vi "WiFi lab coordinator.vi"() -> ()   [LabVIEW 2014]
uses:
  VISA resource XBee.vi
  WiFi API Frame Type.ctl
  WiFi API Frame.ctl
  Protocol enum.ctl
panel:
  out "Port open":bool
  in  "Close serial comm":bool
  in  "Begin serial comm":bool
  in  "VISA resource in":refnum<visa-resource-name>
  out "Link Margin":u32
  out "Channel":u32
  out "Gateway IP":string
  out "Network Mask":string
  out "Destination IP Address":string
  out "Module IP Address":string
  out "Encryption":string
  out "SSID":string
  out "Connection Status":bool
  out "Association Information (AI)":string
  in  "Transparent response string":string
  in  "Transparent control string":string
  in  "Protocol":T1
  in  "Transparent mode enable":bool
  in  "API Response string":string
  in  "API Control string":string
  in  "Start session":bool
  in  "Destination port (hex)":u16=9750 step=1 format="%04x"
  in  "Source port (hex)":u16=2000 step=1 format="%04x"
  out "Source Port":u16
  out "Source IP":u8[](array[numeric])
  out "RF data":string
  # "Serial Port"
  # "Network Information"
  # "Session Configuration"
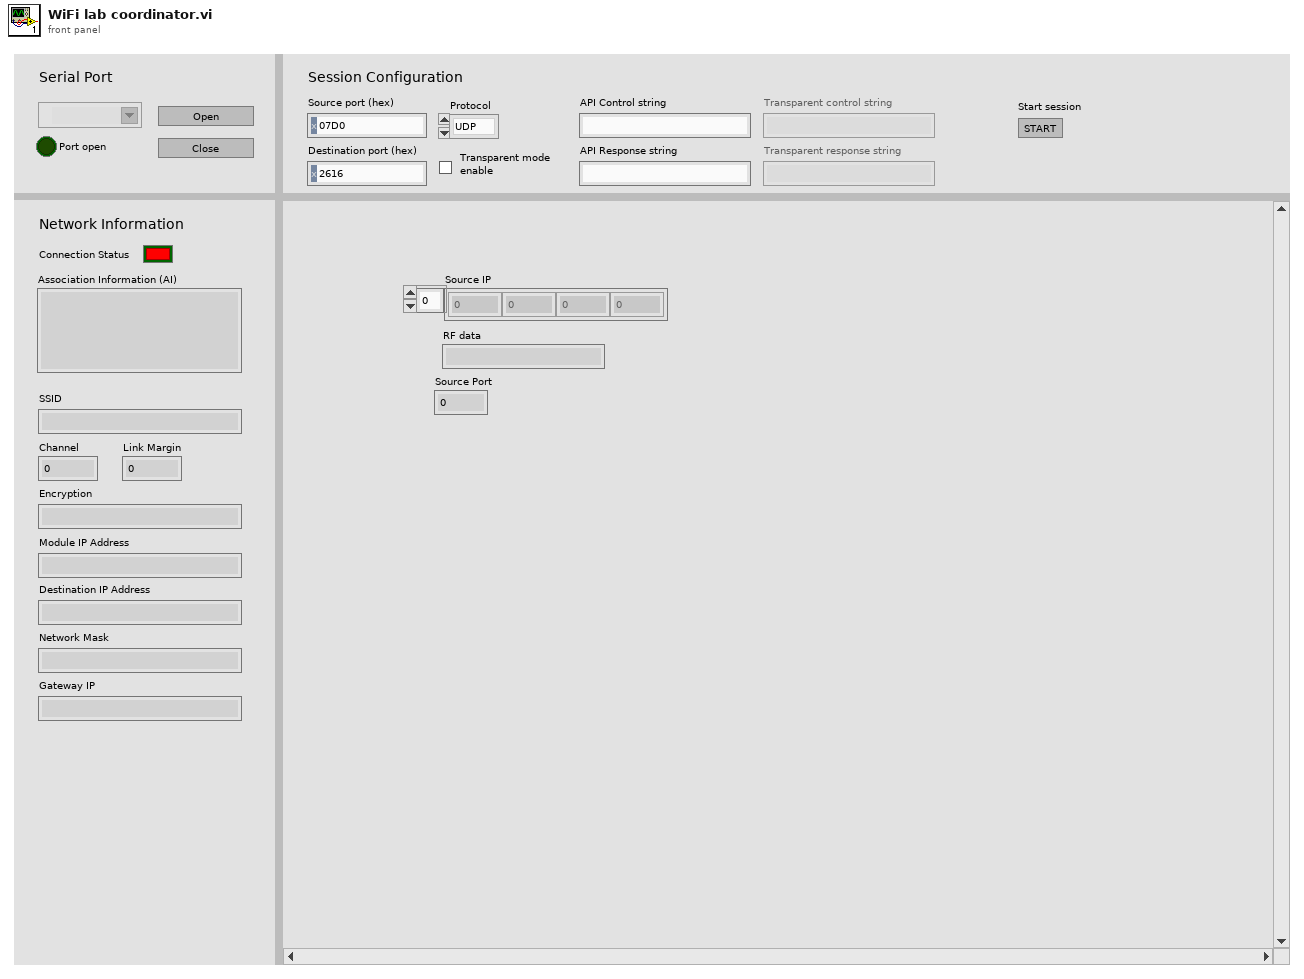
[diagram p1: front panel]
types:
  T1 = typedef "Protocol enum.ctl" = enum8{"UDP", "TCP"}
  T2 = typedef "WiFi API Frame.ctl" = cluster{"Length":u16, "Frame Type":T3, "Payload":u8[], "Checksum":u8}
  T3 = typedef "WiFi API Frame Type.ctl" = u8
  T4 = enum8{"Enabled", "Disabled", "Disabled and Grayed Out"}
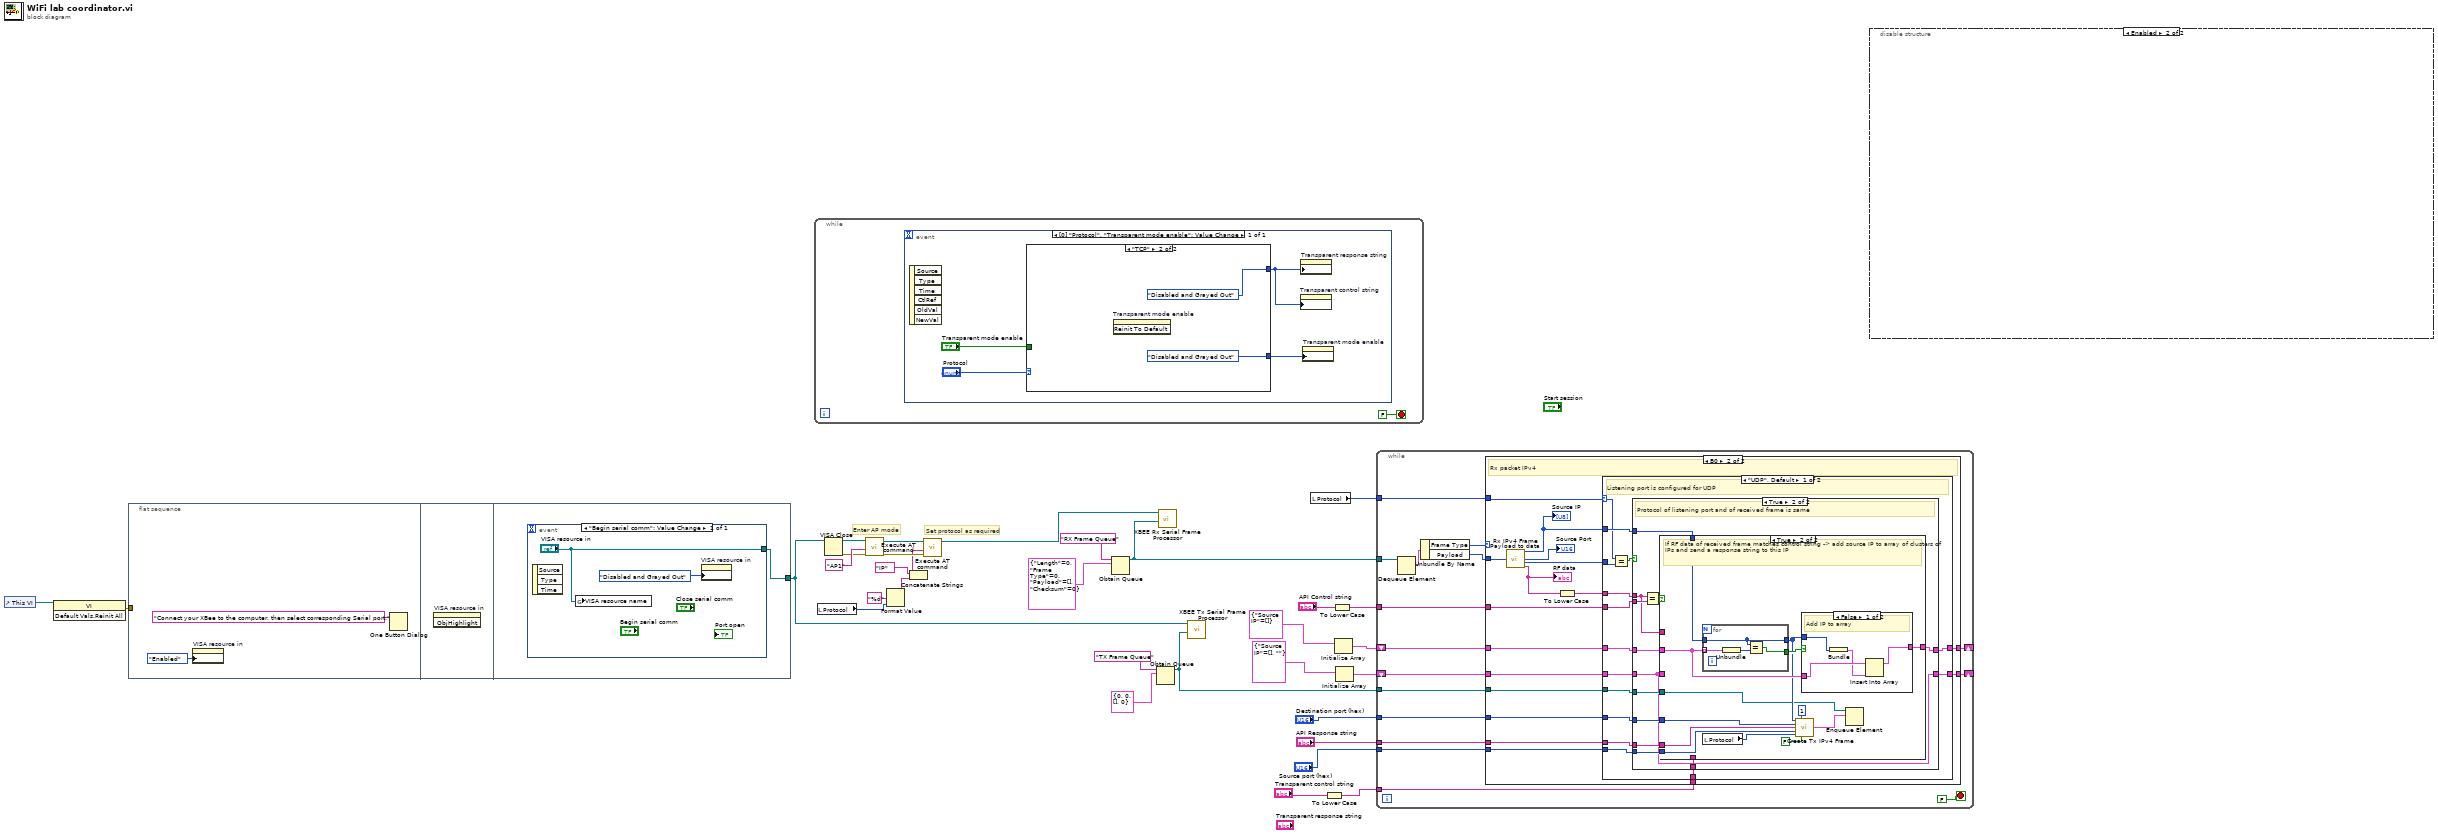
[diagram p0: block diagram]
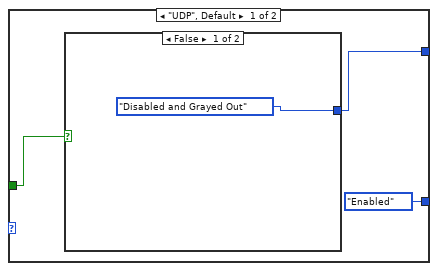
[diagram p2: hidden frame]
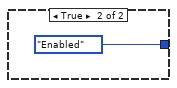
[diagram p3: hidden frame]
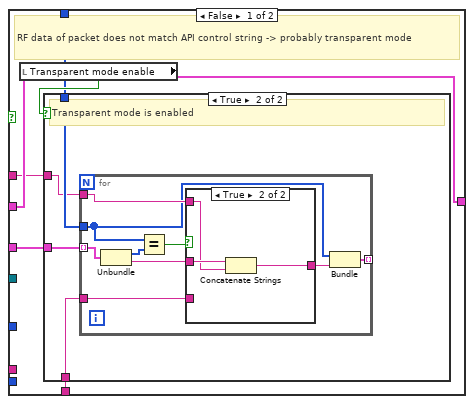
[diagram p6: hidden frame]
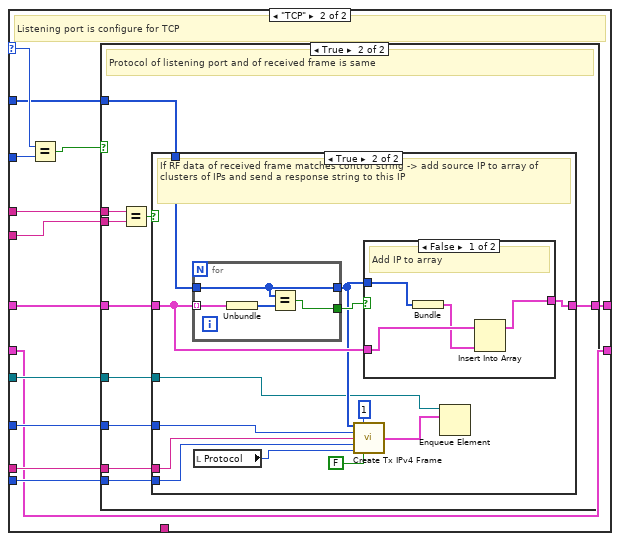
[diagram p10: hidden frame]
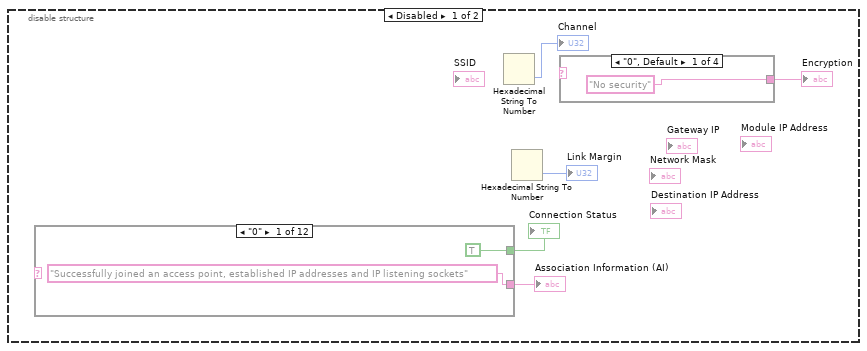
[diagram p14: hidden frame]
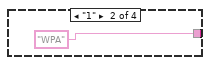
[diagram p15: hidden frame]
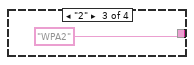
[diagram p16: hidden frame]
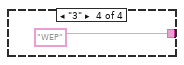
[diagram p17: hidden frame]
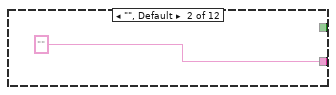
[diagram p18: hidden frame]
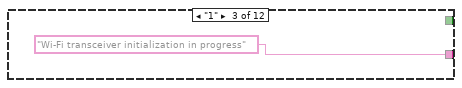
[diagram p19: hidden frame]
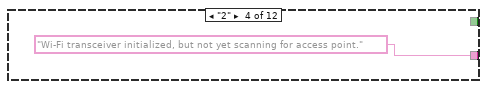
[diagram p20: hidden frame]
diagram:
  # "Set protocol as required"
  # "Enter AP mode"
  n1 = control-ref of="This VI"() -> (w31:refnum<vi>)
  n2 = invoke class="VI" method="Default Vals.Reinit All"(reference=w31) -> (error out=w30:errorcluster)  [unwired: 2 in, 2 out]
  n3 = flat-sequence {
    tunnel: w30 -> [_]
    tunnel: [w34] -> w11
    frame #0 {
      n4 = property on="VISA resource in" class="VISAName"("DisabledEnum"=T4."Enabled" ("Disabled")) -> ()  [unwired: 2 in, 2 out]
      n5 = One Button Dialog(message="Connect your XBee to the computer, then select corresponding Serial port.") -> ()  [unwired: 1 in, 1 out]
    }
    frame #1 {
      n6 = invoke on="VISA resource in" class="VISAName" method="ObjHighlight"() -> ()  [unwired: 3 in, 3 out]
    }
    frame #2 {
      n7 = event shown="[0] \"Begin serial comm\": Value Change" {
        selector: _ -> [_]
        dyn-events: _ -> [_]
        timeout: _ -> [_]
        tunnel: ["VISA resource in"] -> w34
        event "Begin serial comm": Value Change {
          n8 = event-data() -> ()  [unwired: 1 in, 3 out]
          n9 = global write "VISA resource XBee.vi" "VISA resource name"("VISA resource in") -> ()
          n10 = property on="VISA resource in" class="VISAName"("DisabledEnum"=T4."Disabled and Grayed Out" ("Disabled")) -> ()  [unwired: 2 in, 2 out]
        }
      }
    }
  }
  n11 = while {
    stop <- FALSE stop-if-true
    n12 = event shown="[0] \"Protocol\", \"Transparent mode enable\": Value Change" {
      selector: _ -> [_]
      dyn-events: _ -> [_]
      timeout: _ -> [_]
      event "Transparent mode enable": Value Change {
        n13 = event-data() -> ()  [unwired: 1 in, 6 out]
        n14 = case shown="\"TCP\"" "Protocol" {
          tunnel: [T4."Enabled" ("Disabled") T4."Disabled and Grayed Out" ("Disabled")] -> w38
          tunnel: [w42 T4."Disabled and Grayed Out" ("Disabled")] -> w39
          tunnel: "Transparent mode enable" -> [w43 _]
          frame "UDP", Default {
            n15 = case shown="False" w43 {
              tunnel: [T4."Disabled and Grayed Out" ("Disabled") T4."Enabled" ("Disabled")] -> w42
              frame False {
              }
              frame True {
              }
            }
          }
          frame "TCP" {
            n16 = invoke on="Transparent mode enable" class="Bool (strict)" method="Reinit To Default"() -> ()  [unwired: 3 in, 3 out]
          }
        }
        n17 = property on="Transparent control string" class="Str"("DisabledEnum"=w39) -> ()  [unwired: 2 in, 2 out]
        n18 = property on="Transparent response string" class="Str"("DisabledEnum"=w39) -> ()  [unwired: 2 in, 2 out]
        n19 = property on="Transparent mode enable" class="Bool (strict)"("DisabledEnum"=w38) -> ()  [unwired: 2 in, 2 out]
      }
    }
  }
  n20 = local read "Protocol"() -> (w3:T1)
  n21 = VISA Close(VISA resource name=w11) -> (error out=w8:errorcluster)  [unwired: 1 in]
  n22 = call "Execute AT command.vi"("error in (no error)"=w8, "AT Command"="AP1", "VISA resource in"=w11) -> ("error out"=w7:errorcluster, "VISA resource out"=w9:refnum<visa-resource-name>)  [unwired: 5 in, 1 out]
  n23 = Format Value(format string="%d", value (0)=w3) -> (output string=w2:string)  [unwired: 1 in]
  n24 = Concatenate Strings("IP" ("AT Command"), w2) -> (w5:string)
  n25 = call "Execute AT command.vi"("error in (no error)"=w7, "AT Command"=w5, "VISA resource in"=w9) -> ("VISA resource out"=w1:refnum<visa-resource-name>)  [unwired: 5 in, 2 out]
  n26 = Obtain Queue(name (unnamed)="RX Frame Queue", element data type=T2 {"Length"=0, "Frame Type"=0, "Payload"=[], "Checksum"=0} ("API Frame")) -> (queue out=w25:refnum<queue>)  [unwired: 3 in, 2 out]
  n27 = Obtain Queue(name (unnamed)="TX Frame Queue", element data type=T2 {"Length"=0, "Frame Type"=0, "Payload"=[], "Checksum"=0} ("API Frame")) -> (queue out=w19:refnum<queue>)  [unwired: 3 in, 2 out]
  n28 = call "XBEE Rx Serial Frame Processor.vi"("RX Frame Queue"=w25, "VISA Serial Port"=w1) -> ()  [unwired: 8 in, 2 out]
  n29 = call "XBEE Tx Serial Frame Processor.vi"("TX Frame Queue"=w19, "VISA Serial Port"=w11) -> ()  [unwired: 8 in, 2 out]
  n30 = local read "Protocol"() -> (w22:T1)
  n31 = To Lower Case(string="Transparent control string") -> (all lower case string=w12:string)
  n32 = To Lower Case(string="API Control string") -> (all lower case string=w23:string)
  n33 = Initialize Array(cluster{"Source IP":u8[]} {"Source IP"=[]}) -> (w21:cluster{"Source IP":u8[]}[])  [unwired: 1 in]
  n34 = Initialize Array(cluster{"Source IP":u8[], string} {"Source IP"=[], ""}) -> (w14:cluster{"Source IP":u8[], string}[])  [unwired: 1 in]
  n35 = while {
    tunnel: w25 -> [w64]
    tunnel: w23 -> [w59]
    tunnel: w22 -> [w58]
    shift-right: [w55] -> _
    shift-left: w21 -> [w57]
    tunnel: w19 -> [w56]
    tunnel: "Destination port (hex)" -> [w54]
    tunnel: "API Response string" -> [w53]
    tunnel: "Source port (hex)" -> [w52]
    shift-right: [w51] -> _
    shift-left: w14 -> [w49]
    tunnel: w12 -> [w50]
    stop <- FALSE stop-if-true
    n36 = Dequeue Element(queue=w64) -> (element=w63:T2)  [unwired: 2 in, 3 out]
    n37 = Unbundle By Name(w63) -> ("Frame Type"=w62:T3, "Payload"=w61:u8[])
    n38 = case shown="B0" w62 {
      tunnel: w61 -> [_ w83]
      tunnel: w59 -> [_ w78]
      tunnel: w58 -> [_ w80]
      tunnel: w57 -> [w66 w75]
      tunnel: w56 -> [_ w74]
      tunnel: [w66 w73] -> w55
      tunnel: w54 -> [_ w72]
      tunnel: w53 -> [_ w71]
      tunnel: w52 -> [_ w70]
      tunnel: w49 -> [w65 w69]
      tunnel: [w65 w68] -> w51
      tunnel: w50 -> [_ w67]
      frame 0, Default {
      }
      frame 176 {
        # "Rx packet IPv4"
        n39 = call "Rx IPv4 Frame Payload to data.vi"("Payload array"=w83) -> ("Source IP"=w76:u8[], "Source Port"=→"Source Port":u16, "Protocol"=w79:T1, "RF data"=w81:string)  [unwired: 10 in, 1 out]
        "RF data" <- w81
        "Source IP" <- w76
        n40 = To Lower Case(string=w81) -> (all lower case string=w77:string)
        n41 = case shown="\"UDP\", Default" w80 {
          selector: w80 -> [w87 w169]
          tunnel: w79 -> [w88 w170]
          tunnel: w78 -> [w95 w167]
          tunnel: w77 -> [w96 w166]
          tunnel: w76 -> [w90 w165]
          tunnel: w75 -> [w97 w164]
          tunnel: w74 -> [w94 w163]
          tunnel: [w98 w162] -> w73
          tunnel: w72 -> [w93 w161]
          tunnel: w71 -> [w92 w160]
          tunnel: w70 -> [w91 w159]
          tunnel: w69 -> [w86 w158]
          tunnel: [w85 w158] -> w68
          tunnel: w67 -> [w84 _]
          frame "UDP", Default {
            # "Listening port is configured for UDP"
            n42 = Equal?(x=w87, y=w88) -> (x = y?=w89:bool)
            n43 = case shown="True" w89 {
              tunnel: w95 -> [_ w112]
              tunnel: w96 -> [_ w102]
              tunnel: w90 -> [_ w109]
              tunnel: w97 -> [w100 w110]
              tunnel: w94 -> [_ w108]
              tunnel: [w100 w107] -> w98
              tunnel: w93 -> [_ w106]
              tunnel: w92 -> [_ w105]
              tunnel: w91 -> [_ w104]
              tunnel: w86 -> [w99 w103]
              tunnel: [w99 w103] -> w85
              tunnel: w84 -> [_ w101]
              frame False {
                # "Protocol of recieved frame does not match protocol of listening port. \nI know, right?"
              }
              frame True {
                # "Protocol of listening port and of received frame is same"
                n44 = Equal?(x=w102, y=w112) -> (x = y?=w111:bool)
                n45 = case shown="True" w111 {
                  tunnel: w110 -> [w117 w146]
                  tunnel: w109 -> [w115 w148]
                  tunnel: w108 -> [_ w137]
                  tunnel: [w117 w145] -> w107
                  tunnel: w106 -> [_ w143]
                  tunnel: w105 -> [_ w142]
                  tunnel: w104 -> [_ w141]
                  tunnel: w103 -> [w116 _]
                  tunnel: w102 -> [w114 _]
                  tunnel: w101 -> [w113 _]
                  frame False {
                    # "RF data of packet does not match API control string -> probably transparent mode"
                    n46 = local read "Transparent mode enable"() -> (w118:bool)
                    n47 = case shown="True" w118 {
                      tunnel: w116 -> [_ w122]
                      tunnel: w115 -> [_ w121]
                      tunnel: w114 -> [_ w120]
                      tunnel: w113 -> [_ w119]
                      frame False {
                        # "Transparent mode is disabled -> do nothing"
                      }
                      frame True {
                        # "Transparent mode is enabled"
                        n48 = for {
                          tunnel: w122 -> [w131] mode=indexing
                          tunnel: w121 -> [w125]
                          tunnel: w120 -> [w127]
                          tunnel: [w124] -> _ mode=indexing
                          tunnel: w119 -> [w123]
                          n49 = Unbundle(w131) -> ("Source IP"=w130:u8[], w128:string)
                          n50 = Equal?(x=w125, y=w130) -> (x = y?=w129:bool)
                          n51 = case shown="True" w129 {
                            tunnel: w128 -> [w132 w135]
                            tunnel: w127 -> [_ w134]
                            tunnel: [w132 w133] -> w126
                            tunnel: w123 -> [_ _]
                            frame False {
                            }
                            frame True {
                              n52 = Concatenate Strings(w135, w134) -> (w133:string)
                            }
                          }
                          n53 = Bundle("Source IP"=w125, w126) -> (w124:cluster{"Source IP":u8[], string})  [unwired: 1 in]
                        }
                      }
                    }
                  }
                  frame True {
                    # "If RF data of received frame matches control string -> add source IP to array of clusters of IPs and send a response string to this IP"
                    n54 = for {
                      tunnel: w146 -> [w157] mode=indexing
                      tunnel: w148 -> [w154]
                      tunnel: [w155] -> w147
                      tunnel: [w154] -> w144
                      n55 = Unbundle(w157) -> ("Source IP"=w156:u8[])
                      n56 = Equal?(x=w154, y=w156) -> (x = y?=w155:bool)
                    }
                    n57 = local read "Protocol"() -> (w140:T1)
                    n58 = call "Create Tx IPv4 Frame.vi"("Destination IP"=w144, "Frame ID"=u8 1, "Destination port"=w143, "RF data"=w142, "Source port"=w141, "Protocol"=w140, "Transmit options bitfield"=FALSE) -> ("TX IPv4 Frame"=w136:T2)  [unwired: 8 in]
                    n59 = case shown="False" w147 {
                      tunnel: w146 -> [w151 w153]
                      tunnel: w144 -> [w152 _]
                      tunnel: [w149 w153] -> w145
                      frame False {
                        # "Add IP to array"
                        n60 = Bundle("Source IP"=w152) -> (w150:cluster{"Source IP":u8[]})  [unwired: 1 in]
                        n61 = Insert Into Array(array=w151, new element=w150) -> (w149:cluster{"Source IP":u8[]}[])  [unwired: 1 in]
                      }
                      frame True {
                        # "IP already in array"
                      }
                    }
                    n62 = Enqueue Element(queue=w137, element=w136) -> ()  [unwired: 2 in, 3 out]
                  }
                }
              }
            }
          }
          frame "TCP" {
            # "Listening port is configure for TCP"
            n63 = Equal?(x=w169, y=w170) -> (x = y?=w168:bool)
            n64 = case shown="True" w168 {
              tunnel: w167 -> [_ w181]
              tunnel: w166 -> [_ w180]
              tunnel: w165 -> [_ w177]
              tunnel: w164 -> [w171 w178]
              tunnel: w163 -> [_ w176]
              tunnel: [w171 w175] -> w162
              tunnel: w161 -> [_ w174]
              tunnel: w160 -> [_ w173]
              tunnel: w159 -> [_ w172]
              frame False {
                # "Protocol of recieved frame does not match protocol of listening port. \nI know, right?"
              }
              frame True {
                # "Protocol of listening port and of received frame is same"
                n65 = Equal?(x=w180, y=w181) -> (x = y?=w179:bool)
                n66 = case shown="True" w179 {
                  tunnel: w178 -> [w182 w193]
                  tunnel: w177 -> [_ w195]
                  tunnel: w176 -> [_ w184]
                  tunnel: [w182 w192] -> w175
                  tunnel: w174 -> [_ w190]
                  tunnel: w173 -> [_ w189]
                  tunnel: w172 -> [_ w188]
                  frame False {
                    # "RF data of packet does not match control string -> do nothing"
                  }
                  frame True {
                    # "If RF data of received frame matches control string -> add source IP to array of clusters of IPs and send a response string to this IP"
                    n67 = for {
                      tunnel: w193 -> [w204] mode=indexing
                      tunnel: w195 -> [w201]
                      tunnel: [w202] -> w194
                      tunnel: [w201] -> w191
                      n68 = Unbundle(w204) -> ("Source IP"=w203:u8[])
                      n69 = Equal?(x=w201, y=w203) -> (x = y?=w202:bool)
                    }
                    n70 = local read "Protocol"() -> (w187:T1)
                    n71 = call "Create Tx IPv4 Frame.vi"("Destination IP"=w191, "Frame ID"=u8 1, "Destination port"=w190, "RF data"=w189, "Source port"=w188, "Protocol"=w187, "Transmit options bitfield"=FALSE) -> ("TX IPv4 Frame"=w183:T2)  [unwired: 8 in]
                    n72 = case shown="False" w194 {
                      tunnel: w193 -> [w198 w200]
                      tunnel: w191 -> [w199 _]
                      tunnel: [w196 w200] -> w192
                      frame False {
                        # "Add IP to array"
                        n73 = Bundle("Source IP"=w199) -> (w197:cluster{"Source IP":u8[]})  [unwired: 1 in]
                        n74 = Insert Into Array(array=w198, new element=w197) -> (w196:cluster{"Source IP":u8[]}[])  [unwired: 1 in]
                      }
                      frame True {
                        # "IP already in array"
                      }
                    }
                    n75 = Enqueue Element(queue=w184, element=w183) -> ()  [unwired: 2 in, 3 out]
                  }
                }
              }
            }
          }
        }
      }
    }
  }
  n76 = disable-structure shown="Enabled" {
    frame Disabled {
      n77 = case shown="\"0\"" {
        selector: _ -> [_ _ _ _ _ _ _ _ _ _ _ _]
        tunnel: ["Successfully joined an access point, established IP addresses and IP listening sockets" "" "Wi-Fi transceiver initialization in progress" "Wi-Fi transceiver initialized, but not yet scanning for access point." "Disconnecting from access point." "SSID not configured." "Encryption key invalid (either NULL or invalid length for WEP)." "SSID was found, but join failed." "Waiting for WPA or WPA2 Authentication." "Device joined a network and is waiting for IP configuration to complete." "Device is joined, IP is configured, and listening sockets are being set up" "Device is currently scanning for the configured SSID."] -> w209
        tunnel: [TRUE _ _ _ _ _ _ _ _ _ _ _] -> w205
        frame "0" {
        }
        frame "", Default {
        }
        frame "1" {
        }
        frame "2" {
        }
        frame "13" {
        }
        frame "23" {
        }
        frame "24" {
        }
        frame "27" {
        }
        frame "40" {
        }
        frame "41" {
        }
        frame "42" {
        }
        frame "FF" {
        }
      }
      "Association Information (AI)" <- w209
      "Connection Status" <- w205
      n78 = Hexadecimal String To Number() -> (number=→"Channel":u32)  [unwired: 3 in, 1 out]
      n79 = Hexadecimal String To Number() -> (number=→"Link Margin":u32)  [unwired: 3 in, 1 out]
      n80 = case shown="\"0\", Default" {
        selector: _ -> [_ _ _ _]
        tunnel: ["No security" ("format string") "WPA" "WPA2" "WEP"] -> w206
        frame "0", Default {
        }
        frame "1" {
        }
        frame "2" {
        }
        frame "3" {
        }
      }
      "Encryption" <- w206
    }
    frame Enabled {
    }
  }
